vi "SwerveJoystickRotationScaling.vi"(5 "Rotation Maximum":dbl(slide)=1.0 min=0.3 max=1.0 scale=0.3..1.0, 7 "Rotation Scaling":dbl(slide)=2.0 min=1.0 max=4.0 scale=1.0..4.0, 8 "Rotation Deadband":dbl(slide)=0.05 min=0.0 max=0.25 scale=0.0..0.25, 9 "Auto Control":bool, 10 "Raw Joystick Rotation":dbl) -> (0 "Scaled Joystick Rotation":dbl format="%.2f", 2 "In Deadband":bool)   [LabVIEW 2019]
doc: "Applies a deadband and nonlinear scaling to the rotation axis of a swerve drive. Includes a hook to override the non-linear deadband and scaling when the rotation is under autonomous control."
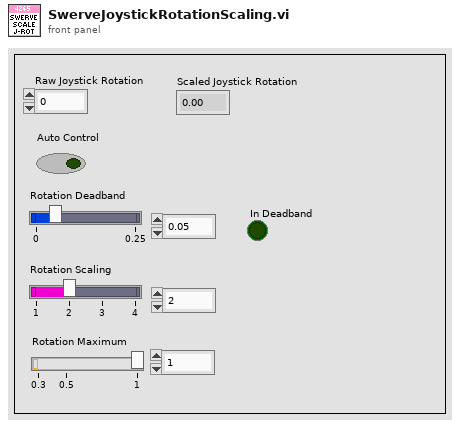
[diagram p1: front panel]
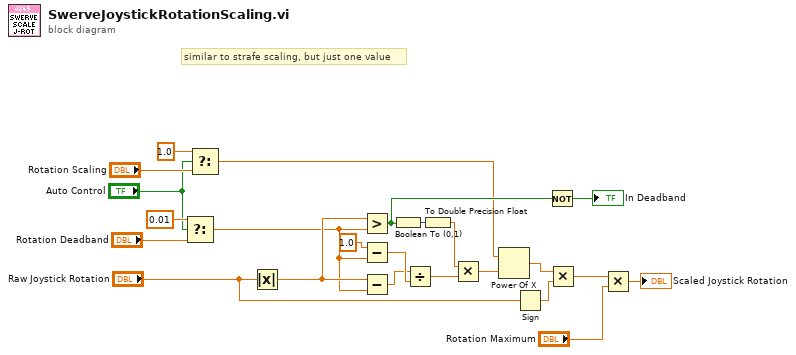
[diagram p0: block diagram]
diagram:
  # "similar to strafe scaling, but just one value"
  n1 = Select(t=0.01, s="Auto Control", f="Rotation Deadband") -> (s? t:f=w9:dbl)
  n2 = Select(t=1.0, s="Auto Control", f="Rotation Scaling") -> (s? t:f=w6:dbl)
  n3 = Absolute Value(x="Raw Joystick Rotation") -> (abs(x)=w19:dbl)
  n4 = Greater?(x=w19, y=w9) -> (0:w20:bool)
  n5 = Subtract(x=1.0, y=w9) -> (x-y=w16:dbl)
  n6 = Subtract(x=w19, y=w9) -> (x-y=w15:dbl)
  n7 = Boolean To (0,1)(Boolean=w20) -> (0, 1=w13:i16)
  n8 = Divide(x=w15, y=w16) -> (x/y=w17:dbl)
  n9 = To Double Precision Float(number=w13) -> (double precision float=w14:dbl)
  n10 = Multiply(x=w14, y=w17) -> (x*y=w22:dbl)
  n11 = Power Of X(1:w22, 2:w6) -> (0:w23:dbl)
  n12 = Sign(1:"Raw Joystick Rotation") -> (0:w18:dbl)
  n13 = Not(x=w20) -> (.not. x?=→"In Deadband":bool)
  n14 = Multiply(x=w23, y=w18) -> (x*y=w3:dbl)
  n15 = Multiply(x=w3, y="Rotation Maximum") -> (x*y=→"Scaled Joystick Rotation":dbl)
